vi "Do Move Teams Array.vi"(7 "Teams in":refnum<class "Team.lvclass">[](array[class]), 8 "Team":i32, 10 "Position":T1, 11 "Square in":refnum<class "Square.lvclass">) -> (3 "Square out":refnum<class "Square.lvclass">, 5 "Teams out":refnum<class "Team.lvclass">[](array[class]))   [LabVIEW 2020, in "SquareBattle.lvlib" / "Square.lvclass"]
uses:
  Square.lvclass
  Square.lvclass/Square.ctl
  Team/Team.lvclass
  Position.ctl
  SquareBattle.lvlib
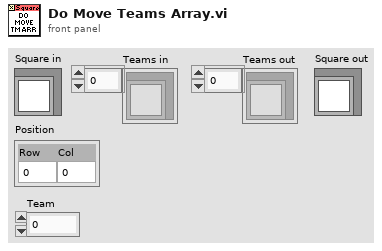
[diagram p1: front panel]
types:
  T1 = typedef "SquareBattle.lvlib/Position.ctl" = cluster{"Row":i32, "Col":i32}
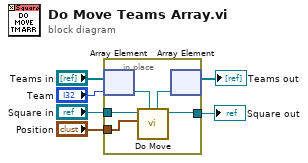
[diagram p0: block diagram]
diagram:
  n1 = in-place {
    in-place-border: "Square in" -> [w11]
    in-place-border: "Position" -> [w10]
    in-place-border: [w7] -> w1
    n2 = in-place-array #1("Teams in", "Team") -> (w9:refnum<class "Team.lvclass">)
    n3 = call "Do Move.vi"("Team in"=w9, "Position"=w10, "Square in"=w11) -> ("Square out"=w7:refnum<class "Square.lvclass">, "Team out"=w8:refnum<class "Team.lvclass">)  [unwired: 7 in]
    n4 = in-place-array #1(w8) -> (→"Teams out":refnum<class "Team.lvclass">[])  [unwired: 1 out]
  }
  "Square out" <- w1
